vi "photometric acquisitions.vi"(8 "error in (no error)":errorcluster, 11 "S4GEI in":refnum<class "S4GEI.lvclass">) -> (0 "error out":errorcluster, 3 "S4GEI out":refnum<class "S4GEI.lvclass">)   [LabVIEW 2018, in "S4GEI.lvclass"]
uses:
  S4GEI.lvclass
  S4GEI.lvclass/S4GEI.ctl
  State Machine/State Machine.lvclass
  Channel GUI/Channel.lvclass
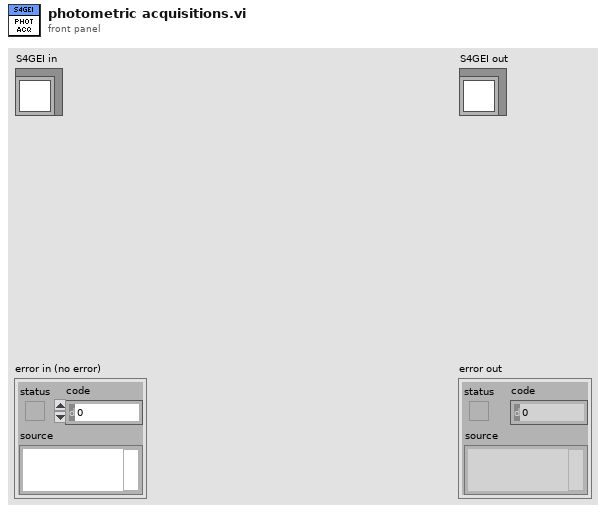
[diagram p1: front panel]
types:
  T1 = cluster{"Acquire":bool, "Stop Acquisition":bool, "Abort Acquisition":bool, "Pause acquisition":bool}
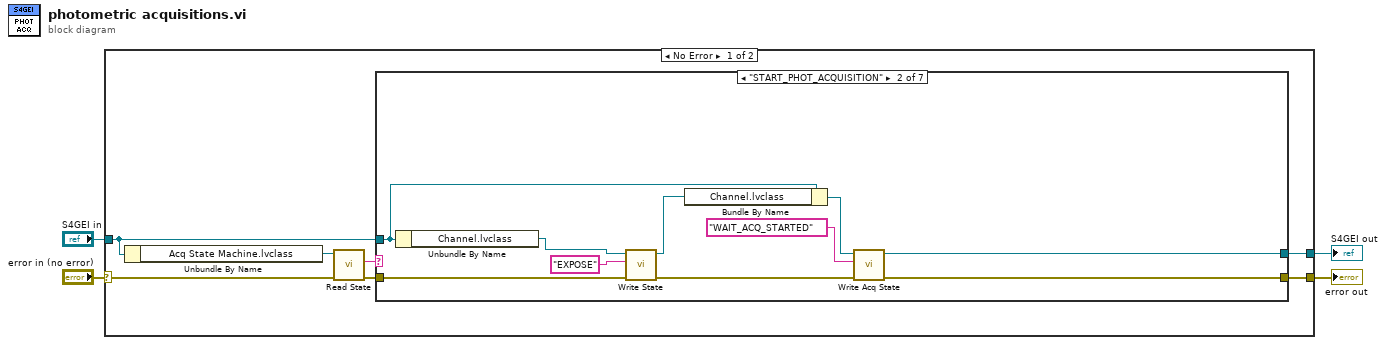
[diagram p0: block diagram]
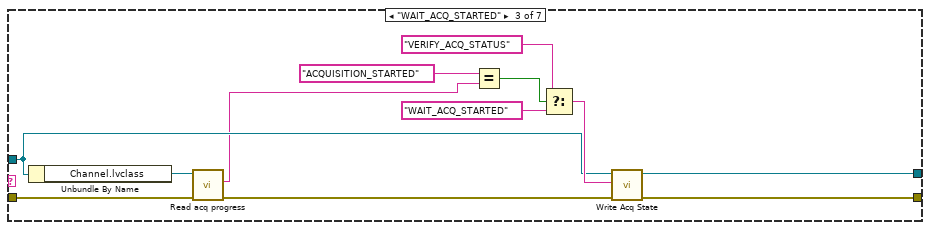
[diagram p3: hidden frame]
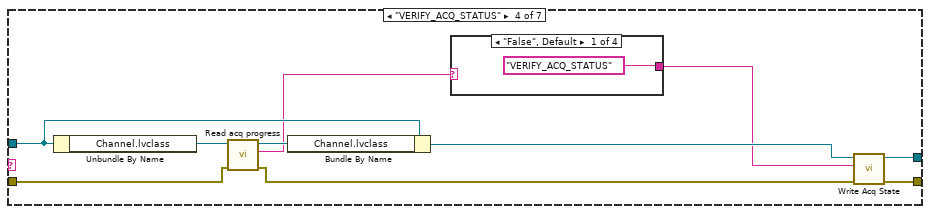
[diagram p4: hidden frame]
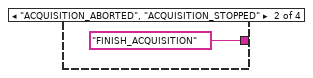
[diagram p5: hidden frame]
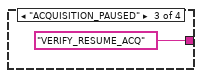
[diagram p6: hidden frame]
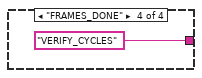
[diagram p7: hidden frame]
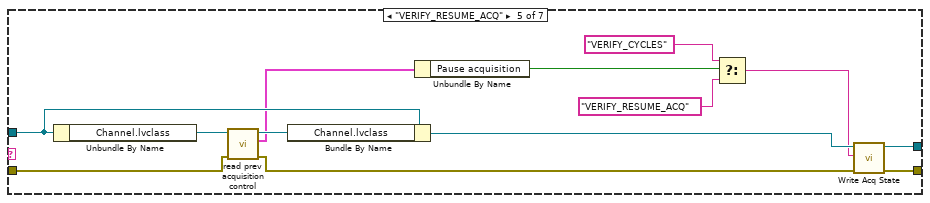
[diagram p8: hidden frame]
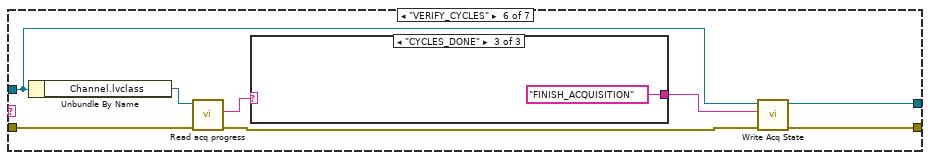
[diagram p9: hidden frame]
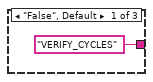
[diagram p10: hidden frame]
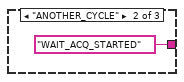
[diagram p11: hidden frame]
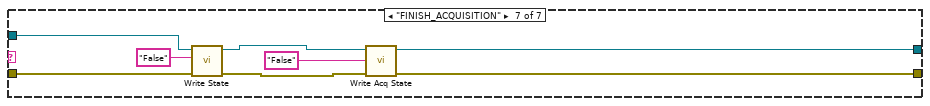
[diagram p12: hidden frame]
diagram:
  n1 = case shown="No Error" "error in (no error)" {
    selector: "error in (no error)" -> [w8 w83]
    tunnel: [w7 w83] -> w3
    tunnel: [w5 w82] -> w1
    tunnel: "S4GEI in" -> [w6 w82]
    frame No Error {
      n2 = Unbundle By Name(w6) -> ("Acq State Machine.lvclass"=w11:refnum<class "State Machine.lvclass">)
      n3 = call-dynamic "Read State.vi"("error in (no error)"=w8, "State Machine in"=w11) -> ("error out"=w9:errorcluster, "State"=w10:string)  [unwired: 7 in, 1 out]
      n4 = case shown="\"START_PHOT_ACQUISITION\"" w10 {
        tunnel: w9 -> [w12 w19 w28 w40 w54 w66 w77]
        tunnel: w6 -> [w13 w16 w30 w45 w60 w68 w78]
        tunnel: [w13 w23 w35 w43 w58 w70 w81] -> w5
        tunnel: [w12 w22 w34 w42 w57 w69 w80] -> w7
        frame "False", Default {
        }
        frame "START_PHOT_ACQUISITION" {
          n5 = Unbundle By Name(w16) -> ("Channel.lvclass"=w20:refnum<class "Channel.lvclass">)
          n6 = call "Write State.vi"("error in (no error)"=w19, "State"="EXPOSE", "Channel GEI in"=w20) -> ("error out"=w17:errorcluster, "Channel GEI out"=w14:refnum<class "Channel.lvclass">)  [unwired: 7 in]
          n7 = Bundle By Name(cluster=w16, "Channel.lvclass"=w14) -> (w15:refnum<class "S4GEI.lvclass">)
          n8 = call "Write Acq State.vi"("error in (no error)"=w17, "State"="WAIT_ACQ_STARTED" ("x"), "SPARC4_GEI in"=w15) -> ("error out"=w22:errorcluster, "SPARC4_GEI out"=w23:refnum<class "S4GEI.lvclass">)  [unwired: 7 in]
        }
        frame "WAIT_ACQ_STARTED" {
          n9 = Unbundle By Name(w30) -> ("Channel.lvclass"=w29:refnum<class "Channel.lvclass">)
          n10 = call-dynamic "Read acq progress.vi"("error in (no error)"=w28, "Channel in"=w29) -> ("error out"=w27:errorcluster, "acq progress"=w26:string)  [unwired: 7 in, 1 out]
          n11 = Equal?(x="ACQUISITION_STARTED" ("State"), y=w26) -> (x = y?=w24:bool)
          n12 = Select(t="VERIFY_ACQ_STATUS" ("State"), s=w24, f="WAIT_ACQ_STARTED" ("State")) -> (s? t:f=w33:string)
          n13 = call "Write Acq State.vi"("error in (no error)"=w27, "State"=w33, "SPARC4_GEI in"=w30) -> ("error out"=w34:errorcluster, "SPARC4_GEI out"=w35:refnum<class "S4GEI.lvclass">)  [unwired: 7 in]
        }
        frame "VERIFY_ACQ_STATUS" {
          n14 = Unbundle By Name(w45) -> ("Channel.lvclass"=w41:refnum<class "Channel.lvclass">)
          n15 = call-dynamic "Read acq progress.vi"("error in (no error)"=w40, "Channel in"=w41) -> ("error out"=w38:errorcluster, "acq progress"=w37:string, "Channel out"=w39:refnum<class "Channel.lvclass">)  [unwired: 7 in]
          n16 = Bundle By Name(cluster=w45, "Channel.lvclass"=w39) -> (w44:refnum<class "S4GEI.lvclass">)
          n17 = case shown="\"False\", Default" w37 {
            tunnel: ["VERIFY_ACQ_STATUS" "FINISH_ACQUISITION" "VERIFY_RESUME_ACQ" "VERIFY_CYCLES"] -> w36
            frame "False", Default {
            }
            frame "ACQUISITION_ABORTED", "ACQUISITION_STOPPED" {
            }
            frame "ACQUISITION_PAUSED" {
            }
            frame "FRAMES_DONE" {
            }
          }
          n18 = call "Write Acq State.vi"("error in (no error)"=w38, "State"=w36, "SPARC4_GEI in"=w44) -> ("error out"=w42:errorcluster, "SPARC4_GEI out"=w43:refnum<class "S4GEI.lvclass">)  [unwired: 7 in]
        }
        frame "VERIFY_RESUME_ACQ" {
          n19 = Unbundle By Name(w60) -> ("Channel.lvclass"=w55:refnum<class "Channel.lvclass">)
          n20 = call-dynamic "read prev acquisition control.vi"("error in (no error)"=w54, "Channel in"=w55) -> ("error out"=w52:errorcluster, "prev acquisition control"=w51:T1, "Channel out"=w53:refnum<class "Channel.lvclass">)  [unwired: 7 in]
          n21 = Bundle By Name(cluster=w60, "Channel.lvclass"=w53) -> (w59:refnum<class "S4GEI.lvclass">)
          n22 = Unbundle By Name(w51) -> ("Pause acquisition"=w50:bool)
          n23 = Select(t="VERIFY_CYCLES", s=w50, f="VERIFY_RESUME_ACQ") -> (s? t:f=w56:string)
          n24 = call "Write Acq State.vi"("error in (no error)"=w52, "State"=w56, "SPARC4_GEI in"=w59) -> ("error out"=w57:errorcluster, "SPARC4_GEI out"=w58:refnum<class "S4GEI.lvclass">)  [unwired: 7 in]
        }
        frame "VERIFY_CYCLES" {
          n25 = Unbundle By Name(w68) -> ("Channel.lvclass"=w67:refnum<class "Channel.lvclass">)
          n26 = call-dynamic "Read acq progress.vi"("error in (no error)"=w66, "Channel in"=w67) -> ("error out"=w65:errorcluster, "acq progress"=w64:string)  [unwired: 7 in, 1 out]
          n27 = case shown="\"CYCLES_DONE\"" w64 {
            tunnel: ["VERIFY_CYCLES" ("State") "WAIT_ACQ_STARTED" ("y") "FINISH_ACQUISITION" ("State")] -> w63
            frame "False", Default {
            }
            frame "ANOTHER_CYCLE" {
            }
            frame "CYCLES_DONE" {
            }
          }
          n28 = call "Write Acq State.vi"("error in (no error)"=w65, "State"=w63, "SPARC4_GEI in"=w68) -> ("error out"=w69:errorcluster, "SPARC4_GEI out"=w70:refnum<class "S4GEI.lvclass">)  [unwired: 7 in]
        }
        frame "FINISH_ACQUISITION" {
          n29 = call "Write State.vi"("error in (no error)"=w77, "State"="False", "SPARC4_GEI in"=w78) -> ("error out"=w76:errorcluster, "SPARC4_GEI out"=w79:refnum<class "S4GEI.lvclass">)  [unwired: 7 in]
          n30 = call "Write Acq State.vi"("error in (no error)"=w76, "State"="False", "SPARC4_GEI in"=w79) -> ("error out"=w80:errorcluster, "SPARC4_GEI out"=w81:refnum<class "S4GEI.lvclass">)  [unwired: 7 in]
        }
      }
    }
    frame Error {
    }
  }
  "error out" <- w3
  "S4GEI out" <- w1
